vi "DIO (A).vi"(0 "Dio":refnum<k24>, 1 "DIO Status P1 W":bool[](array[boolean]), 4 "DIO Status P2 W":bool[](array[boolean]), 5 "error in (no error)":errorcluster, 6 "Port P1":i32(ring) items=["Port_A", "Port_B", "Port_C"], 7 "Port P2":i32(ring) items=["Port_A", "Port_B", "Port_C"], 8 "P1 Direction":enum16{"Input(read)", "Output(write)"}(ring), 9 "P2 Direction":enum16{"Input(read)", "Output(write)"}(ring)) -> (12 "Disable P1 W":u8=2, 13 "Disable P2 W":u8=2, 14 "DIO Status P1 R":bool[](array[boolean]), 15 "Disable P1 R":u8=2, 17 "DIO Status P2 R":bool[](array[boolean]), 18 "Disable P2 R":u8=2, 19 "error out":errorcluster)   [LabVIEW 2011]
doc: "Control the digital input/output port manually(advanced version)."
uses:
  C:/Program Files/Metrohm Autolab/Autolab SDK 1.10/EcoChemie.Autolab.Sdk.dll
  EcoChemie.Autolab.Sdk.dll
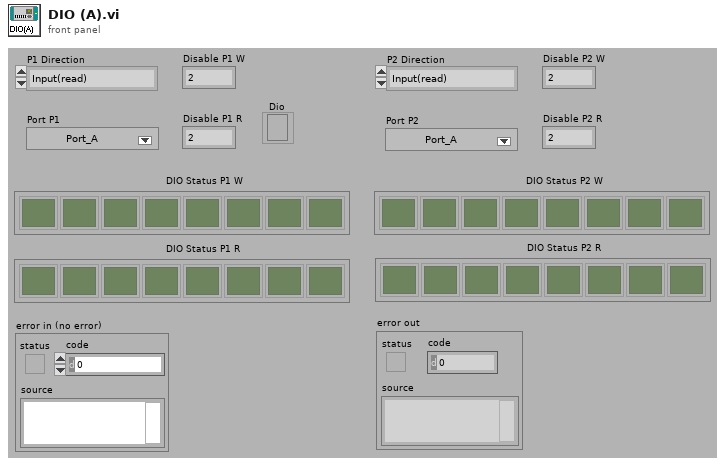
[diagram p1: front panel]
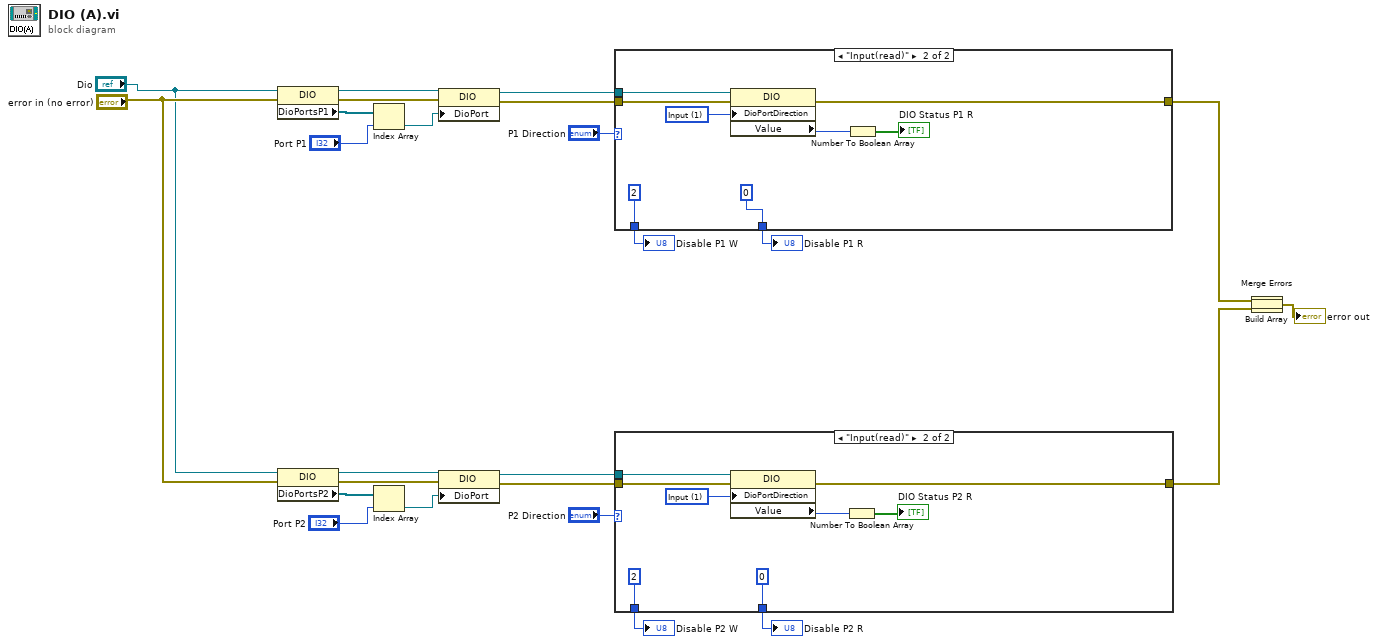
[diagram p0: block diagram]
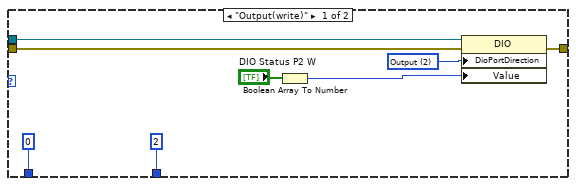
[diagram p2: hidden frame]
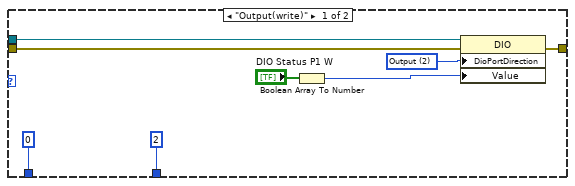
[diagram p3: hidden frame]
diagram:
  n1 = property class="DIO"(reference="Dio", error in="error in (no error)") -> (reference out=w26:refnum<k24>, error out=w25:errorcluster, "DioPortsP1"=w23:refnum<k24>[])
  n2 = property class="DIO"(reference="Dio", error in="error in (no error)") -> (reference out=w18:refnum<k24>, error out=w17:errorcluster, "DioPortsP2"=w15:refnum<k24>[])
  n3 = Index Array(array=w23, index="Port P1") -> (element=w24:refnum<k24>)
  n4 = Index Array(array=w15, index="Port P2") -> (element=w16:refnum<k24>)
  n5 = property class="DIO"(reference=w26, error in=w25, "DioPort"=w24) -> (reference out=w22:refnum<k24>, error out=w21:errorcluster)
  n6 = property class="DIO"(reference=w18, error in=w17, "DioPort"=w16) -> (reference out=w14:refnum<k24>, error out=w13:errorcluster)
  n7 = case shown="\"Input(read)\"" "P1 Direction" {
    tunnel: w22 -> [w33 w41]
    tunnel: w21 -> [w32 w40]
    tunnel: [w31 w39] -> w9
    tunnel: [u8 0 ("Disabled") u8 2 ("Disabled")] -> w6
    tunnel: [u8 2 ("Disabled") u8 0 ("Disabled")] -> w5
    frame "Output(write)" {
      w34 = u8 2 items=["Input"=1, "Output"=2] ("DioPortDirection")
      n8 = Boolean Array To Number(Boolean array="DIO Status P1 W") -> (number=w29:u32)
      n9 = property class="DIO"(reference=w33, error in=w32, "DioPortDirection"=w34, "Value"=w29) -> (error out=w31:errorcluster)  [unwired: 1 out]
    }
    frame "Input(read)" {
      w42 = u8 1 items=["Input"=1, "Output"=2] ("DioPortDirection")
      n10 = property class="DIO"(reference=w41, error in=w40, "DioPortDirection"=w42) -> (error out=w39:errorcluster, "Value"=w37:u8)  [unwired: 1 out]
      n11 = Number To Boolean Array(number=w37) -> (Boolean array=→"DIO Status P1 R":bool[])
    }
  }
  "Disable P1 W" <- w6
  "Disable P1 R" <- w5
  n12 = case shown="\"Input(read)\"" "P2 Direction" {
    tunnel: w14 -> [w49 w57]
    tunnel: w13 -> [w48 w56]
    tunnel: [w47 w55] -> w8
    tunnel: [u8 0 ("Disabled") u8 2 ("Disabled")] -> w4
    tunnel: [u8 2 ("Disabled") u8 0 ("Disabled")] -> w3
    frame "Output(write)" {
      w50 = u8 2 items=["Input"=1, "Output"=2] ("DioPortDirection")
      n13 = Boolean Array To Number(Boolean array="DIO Status P2 W") -> (number=w45:u32)
      n14 = property class="DIO"(reference=w49, error in=w48, "DioPortDirection"=w50, "Value"=w45) -> (error out=w47:errorcluster)  [unwired: 1 out]
    }
    frame "Input(read)" {
      w58 = u8 1 items=["Input"=1, "Output"=2] ("DioPortDirection")
      n15 = property class="DIO"(reference=w57, error in=w56, "DioPortDirection"=w58) -> (error out=w55:errorcluster, "Value"=w53:u8)  [unwired: 1 out]
      n16 = Number To Boolean Array(number=w53) -> (Boolean array=→"DIO Status P2 R":bool[])
    }
  }
  "Disable P2 W" <- w4
  "Disable P2 R" <- w3
  n17 = Build Array(w9, w8) -> (w1:errorcluster[])
  n18 = Merge Errors(w1) -> (→"error out":errorcluster)
